vi "Main.vi"() -> ()   [LabVIEW 2018]
uses:
  <vilib>/MakerHub/LINX/Public/Peripherals/PWM/PWM Set Duty Cycle 1 Chan.vi
  <vilib>/MakerHub/LINX/Public/Utilities/Open Serial.vi
  <vilib>/MakerHub/LINX/Public/Peripherals/PWM/PWM Set Duty Cycle N Chans.vi
  <vilib>/MakerHub/LINX/LMH-LINX.lvlib
panel:
  in  "Speed RPM":dbl(knob) scale=-100.0..100.0
  in  "Baud Rate":u32=9600
  in  "?":bool
  out "error out":errorcluster
  in  "Serial Port":refnum<visa-resource-name>="N/A"
  # "Arduino Settings"
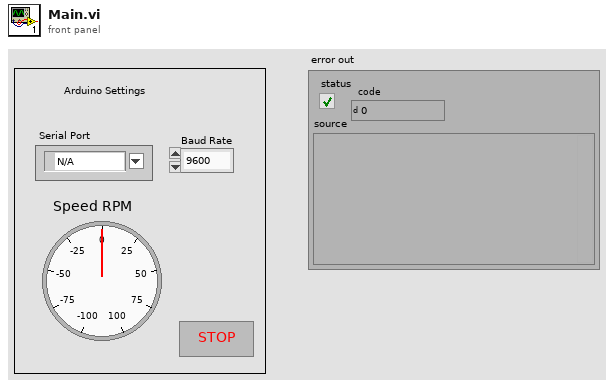
[diagram p1: front panel]
types:
  T1 = typedef "LMH-LINX.lvlib/LINX Ref.ctl" = cluster{"IO":T2, "Interface":T3, "LINX Device Config":T4}
  T2 = typedef "LMH-LINX.lvlib/Platform.ctl" = enum16{"Remote", "Local"}
  T3 = typedef "LMH-LINX.lvlib/Interface.ctl" = enum16{"Serial", "TCP"}
  T4 = typedef "LMH-LINX.lvlib/Device.lvlib/LINX Device Config.ctl" = cluster{"Interface":T3, "COM Port":refnum<visa-resource-name>, "TCP Configuration":T5, "Device Family":u8, "Device ID":u8, "Device Name":string, "TCP Ref":refnum<k5>, "Channels":T6}
  T5 = typedef "LMH-LINX.lvlib/Device.lvlib/TCP Config.ctl" = cluster{"IP Address":string, "Port":u16}
  T6 = typedef "LMH-LINX.lvlib/Channels.ctl" = cluster{"DI":u8[], "DO":u8[], "AI":u8[], "AO":u8[], "PWM":u8[], "QE":u8[], "UART":u8[], "I2C 2":u8[], "SPI":u8[], "CAN":u8[], "Servo":u8[], "AI Ref (V)":dbl, "AI Resolution (Bits)":u8, "AO Ref (V)":dbl, "AO Resolution (Bits)":u8}
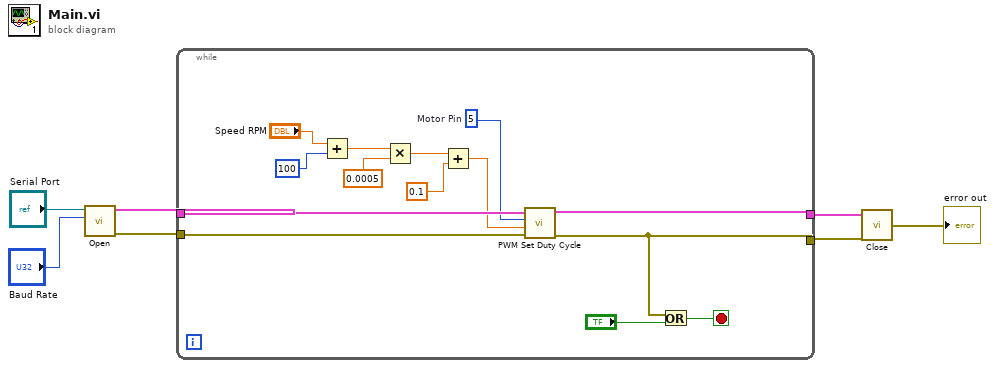
[diagram p0: block diagram]
diagram:
  n1 = call-poly <vilib>:"Open.vi"("Baud Rate Override"="Baud Rate", "Serial Port"="Serial Port") -> ("Error Out"=w3:errorcluster, "LINX Resource"=w4:T1)  [unwired: 7 in, 1 out]
  n2 = while {
    tunnel: w4 -> [w21]
    tunnel: w3 -> [w19]
    tunnel: [w20] -> w2
    tunnel: [w16] -> w1
    stop <- w15 stop-if-true
    w18 = u8 5  # Motor Pin
    n3 = Add(x="Speed RPM", y=100) -> (x+y=w13:dbl)
    n4 = Multiply(x=w13, y=0.0005) -> (x*y=w14:dbl)
    n5 = Add(x=w14, y=0.1) -> (x+y=w8:dbl)
    n6 = call-poly <vilib>:"PWM Set Duty Cycle.vi"("Error In"=w19, "Duty Cycle (0-1)"=w8, "PWM Channel"=w18, "LINX Resource"=w21) -> ("Error Out"=w16:errorcluster, "LINX Resource"=w20:T1)  [unwired: 6 in]
    n7 = Or(x=w16, y="?") -> (x .or. y?=w15:bool)
  }
  n8 = call <vilib>:"Close.vi"("Error In"=w1, "LINX Resource"=w2) -> ("Error Out"=→"error out":errorcluster)  [unwired: 9 in]
